vi "Query.vi"(8 "error in":errorcluster, 10 "Query":string, 11 "DB-Engine in":refnum<class "DB-Interface.lvclass">) -> (0 "error out":errorcluster, 1 "Meta Data":variant, 2 "Return Data":string[][](array[string]), 3 "DB-Engine out":refnum<class "DB-Interface.lvclass">, 4 "Field Names":string[](array[string]))   [LabVIEW 2020, in "hse-db.lvlib" / "DB-Interface.lvclass"]
doc: "____\nHAMPEL SOFTWARE ENGINEERING v1.4.0 (2023-12-19 09:52)"
uses:
  DB-Interface.lvclass
  DB-Interface.lvclass/DB-Interface.ctl
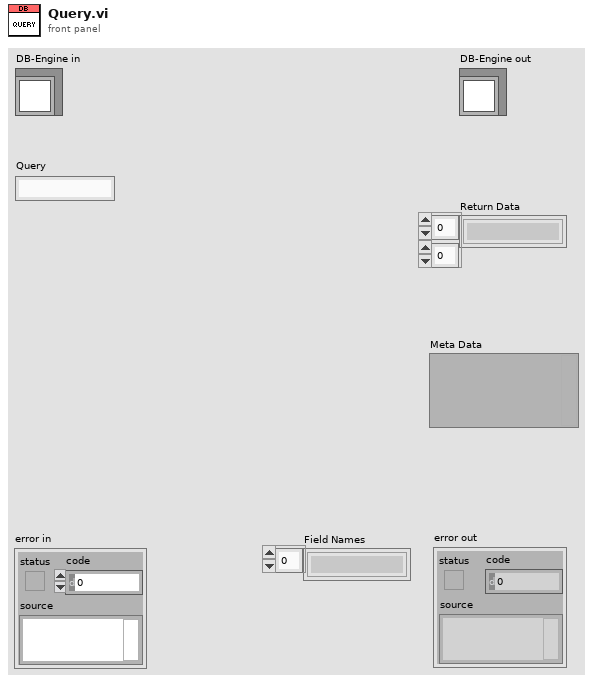
[diagram p1: front panel]
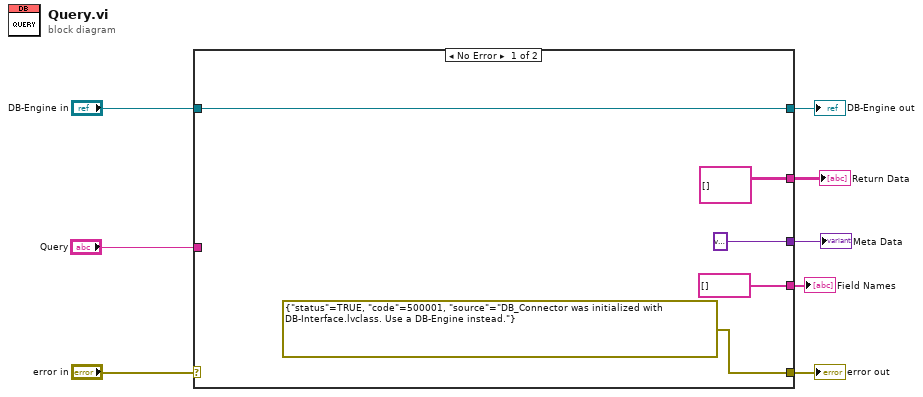
[diagram p0: block diagram]
diagram:
  n1 = case shown="No Error" "error in" {
    selector: "error in" -> [_ w15]
    tunnel: [errorcluster {"status"=TRUE, "code"=500001, "source"="DB_Connector was initialized with DB-Interface.lvclass. Use a DB-Engine instead."} ("error IO") w15] -> w7
    tunnel: [w13 w14] -> w5
    tunnel: "DB-Engine in" -> [w13 w14]
    tunnel: "Query" -> [_ _]
    tunnel: [string[][] [] _] -> w2
    tunnel: [variant _] -> w3
    tunnel: [string[] [] _] -> w1
    frame No Error {
    }
    frame Error {
    }
  }
  "error out" <- w7
  "DB-Engine out" <- w5
  "Meta Data" <- w3
  "Return Data" <- w2
  "Field Names" <- w1
